vi "Start et Init Cam.vi"(8 "error in (no error)":errorcluster caption="entrée d'erreur (pas d'erreur)", 10 "Session In":T1, 11 "Acq Cam Basler en entrée":refnum<class "Acq Cam Basler.lvclass">) -> (0 "error out":errorcluster caption="sortie d'erreur", 2 "Session Out":T1, 3 "Acq Cam Basler en sortie":refnum<class "Acq Cam Basler.lvclass">)   [LabVIEW 2023, in "Acq Cam Basler.lvclass"]
uses:
  Acq Cam Basler.lvclass
  C:/Program Files (x86)/National Instruments/LabVIEW 2023/vi.lib/addons/_Workers/Library/Classes/Worker/Worker.lvclass
  <vilib>/userDefined/High Color/IMAQdx.ctl
  <vilib>/vision/driver/IMAQdx.llb/IMAQdx Acquisition Mode.ctl
  <vilib>/vision/driver/IMAQdx.llb/IMAQdx Camera Control Mode.ctl
  Acq Cam Basler.lvclass/Acq Cam Basler.ctl
  <vilib>/addons/_Workers/Library/Classes/Message/Enqueue Message to Queue.vi
  <vilib>/vision/driver/NI_Vision_Acquisition_Software.lvlib
  <resource>/objmgr/imaqdx.rc
  <vilib>/addons/_Workers/Library/Classes/Message/Message.lvclass
  UI Cam Basler/UI Cam Basler.lvclass
  C:/Program Files (x86)/National Instruments/LabVIEW 2023/vi.lib/addons/_Workers/Library/Classes/Workers Object/Workers Object.lvclass
  C:/Users/flepetit/Desktop/CamView-mdi-LV/Workers/Acq Cam Basler/Acq Cam Basler.lvclass
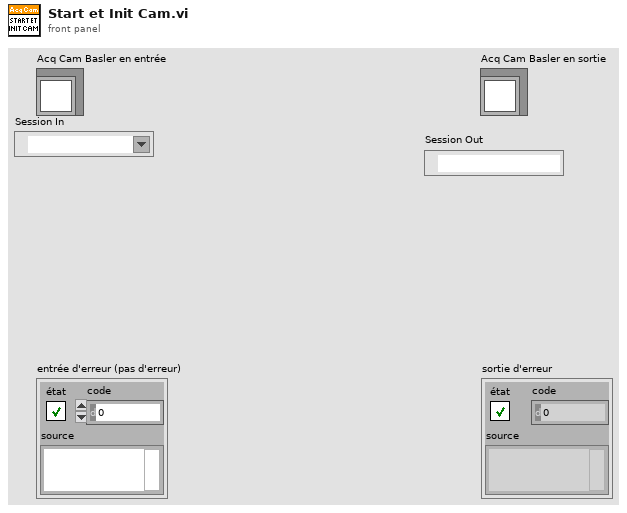
[diagram p1: front panel]
types:
  T1 = typedef "IMAQdx.ctl" = refnum<k21>
  T2 = typedef "NI_Vision_Acquisition_Software.lvlib/IMAQdx Camera Control Mode.ctl" = enum32{"Controller", "Listener"}
  T3 = typedef "NI_Vision_Acquisition_Software.lvlib/IMAQdx Acquisition Mode.ctl" = enum32{"One Shot", "Continuous"}
  T4 = typedef "Image Type" = u32
  T5 = typedef "IMAQ Image.ctl" = refnum<image>
  T6 = typedef "Workers.lvlib/Case Label.ctl" = string
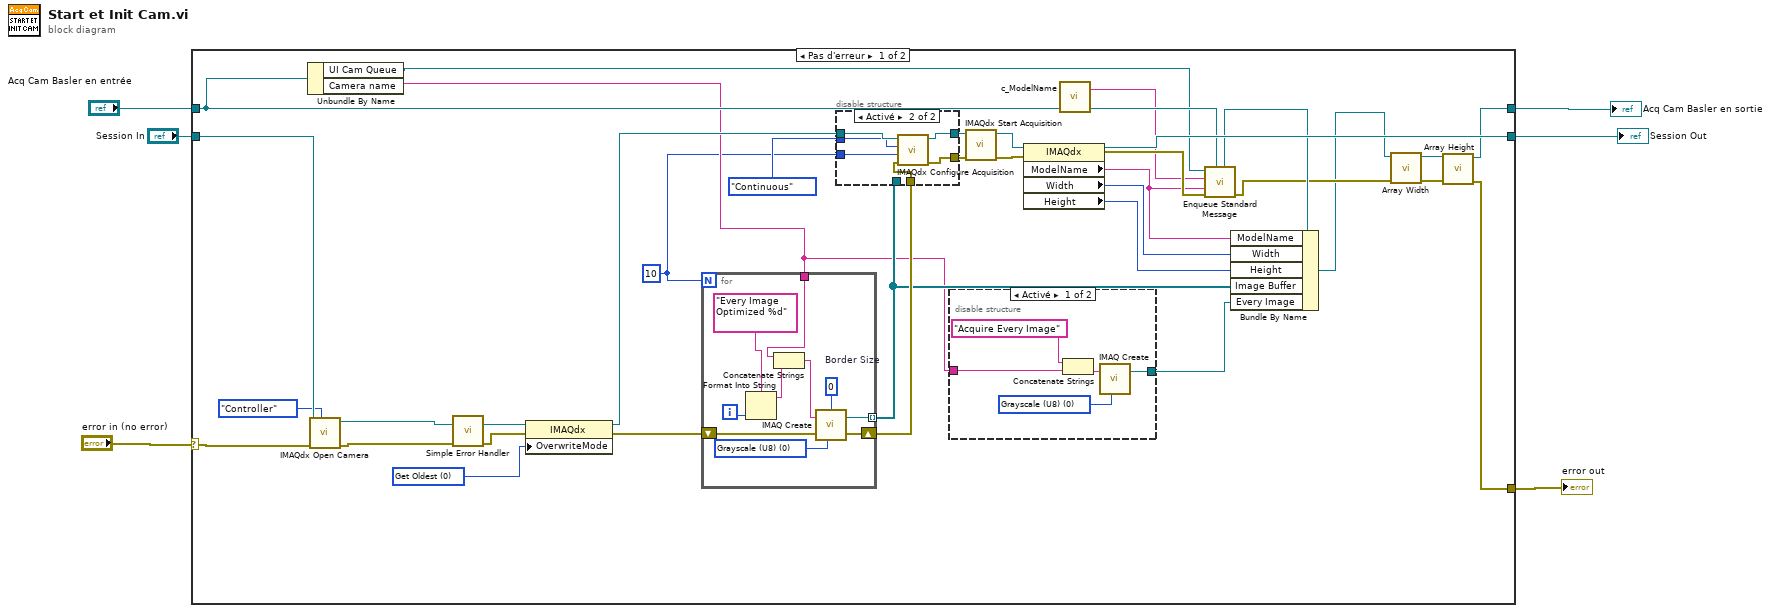
[diagram p0: block diagram]
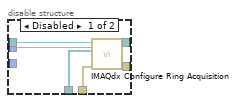
[diagram p3: hidden frame]
diagram:
  n1 = case shown="Pas d'erreur" "error in (no error)" {
    selector: "error in (no error)" -> [w33 w70]
    tunnel: [w9 w70] -> w5
    tunnel: [w7 w69] -> w3
    tunnel: "Acq Cam Basler en entrée" -> [w27 w69]
    tunnel: [w29 w68] -> w2
    tunnel: "Session In" -> [w32 w68]
    frame No Error {
      w13 = 10 ("Number of Images")
      w14 = u16 0 items=["Get Oldest"=0, "Fail"=2, "Get Newest"=3] ("Overwrite Mode")
      n2 = Unbundle By Name(w27) -> ("UI Cam Queue"=w24:refnum<class "Message Queue.lvclass">, "Camera name"=w15:string)
      n3 = call <vilib>:"IMAQdx Open Camera.vi"("Camera Control Mode"=IMAQdx_Camera_Control_Mode."Controller", "error in"=w33, "Session In"=w32) -> ("error out"=w20:errorcluster, "Session Out"=w36:T1)  [unwired: 7 out]
      n4 = call <vilib>:"Simple Error Handler.vi"("error in (no error)"=w20) -> ("error out"=w19:errorcluster)  [unwired: 4 in, 4 out]
      n5 = property class="IMAQdx"(reference=w36, error in=w19, "OverwriteMode"=w14) -> (reference out=w35:T1, error out=w34:errorcluster)
      n6 = for {
        N: w13 -> [_]
        tunnel: [w62] -> w31 mode=indexing
        shift-right: [w66] -> w38
        shift-left: w34 -> [w67]
        tunnel: w15 -> [w60]
        i -> [w65]
        w58 = T4 0 items=["Grayscale (U8)", "Grayscale (I16)", "Grayscale (SGL)", "Complex (CSG)", "RGB (U32)", "HSL (U32)", "RGB (U64)", "Grayscale (U16)"] ("Image Type")
        w63 = 0  # Border Size
        n7 = Format Into String(format string="Every Image Optimized %d" ("Image Name"), w65) -> (resulting string=w61:string)  [unwired: 2 in, 1 out]
        n8 = Concatenate Strings(w60, w61) -> (w59:string)
        n9 = call "IMAQ Create"("Border Size"=w63, "Image Name"=w59, "Image Type"=w58, "error in (no error)"=w67) -> ("New Image"=w62:T5, "error out"=w66:errorcluster)  [unwired: 1 out]
      }
      n10 = disable-structure shown="Activé" {
        disable-tunnel: [w51 w56] -> w40
        disable-tunnel: [w50 w55] -> w39
        disable-tunnel: w38 -> [w49 w54]
        disable-tunnel: IMAQdx_Acquisition_Mode."Continuous" ("Continuous?") -> [w48 w52]
        disable-tunnel: w35 -> [w47 w57]
        disable-tunnel: w31 -> [w46 _]
        disable-tunnel: w13 -> [_ w53]
        frame Disabled {
          n11 = call <vilib>:"IMAQdx Configure Ring Acquisition.vi"("Mode"=w48, "error in"=w49, "Images"=w46, "Session In"=w47) -> ("error out"=w50:errorcluster, "Session Out"=w51:T1)  [unwired: 5 in, 1 out]
        }
        frame Enabled {
          n12 = call <vilib>:"IMAQdx Configure Acquisition.vi"("error in"=w54, "Number of Buffers"=w53, "Continuous?"=w52, "Session In"=w57) -> ("error out"=w55:errorcluster, "Session Out"=w56:T1)  [unwired: 6 in]
        }
      }
      n13 = disable-structure shown="Activé" {
        disable-tunnel: [w45 _] -> w16
        disable-tunnel: w15 -> [w42 _]
        frame Enabled {
          w44 = T4 0 items=["Grayscale (U8)", "Grayscale (I16)", "Grayscale (SGL)", "Complex (CSG)", "RGB (U32)", "HSL (U32)", "RGB (U64)", "Grayscale (U16)"] ("Image Type")
          n14 = Concatenate Strings("Acquire Every Image" ("Image Name"), w42) -> (w41:string)
          n15 = call "IMAQ Create"("Image Name"=w41, "Image Type"=w44) -> ("New Image"=w45:T5)  [unwired: 2 in, 2 out]
        }
        frame Disabled {
        }
      }
      n16 = call <vilib>:"IMAQdx Start Acquisition.vi"("error in"=w39, "Session In"=w40) -> ("error out"=w28:errorcluster, "Session Out"=w30:T1)  [unwired: 8 out]
      n17 = property class="IMAQdx"(reference=w30, error in=w28) -> (reference out=w29:T1, error out=w25:errorcluster, "ModelName"=w22:string, "Width"=w18:u32, "Height"=w17:u32)
      n18 = call "c_ModelName.vi"() -> ("Case Label"=w23:T6)  [unwired: 1 in]
      n19 = call-poly <vilib>:"Enqueue Standard Message.vi"("Worker"=w27, "error in"=w25, "Data"=w22, "Case Label"=w23, "Message Queue"=w24) -> ("error out"=w12:errorcluster, "dup Worker out"=w26:refnum<class "Acq Cam Basler.lvclass">)  [unwired: 4 in, 1 out]
      n20 = Bundle By Name(cluster=w26, "ModelName"=w22, "Width"=w18, "Height"=w17, "Image Buffer"=w31, "Every Image"=w16) -> (w11:refnum<class "Acq Cam Basler.lvclass">)
      n21 = call "Array Width.vi"("error in (no error)"=w12, "Acq Cam Basler en entrée"=w11) -> ("error out"=w10:errorcluster, "Acq Cam Basler en sortie"=w8:refnum<class "Acq Cam Basler.lvclass">)  [unwired: 8 in]
      n22 = call "Array Height.vi"("error in (no error)"=w10, "Acq Cam Basler en entrée"=w8) -> ("error out"=w9:errorcluster, "Acq Cam Basler en sortie"=w7:refnum<class "Acq Cam Basler.lvclass">)  [unwired: 8 in]
    }
    frame Error {
    }
  }
  "error out" <- w5
  "Acq Cam Basler en sortie" <- w3
  "Session Out" <- w2
